vi "IGC100 Close.vi"(2 "error in":errorcluster, 3 "VISA in":refnum<visa-resource-name>) -> (0 "error out":errorcluster)   [LabVIEW 2010]
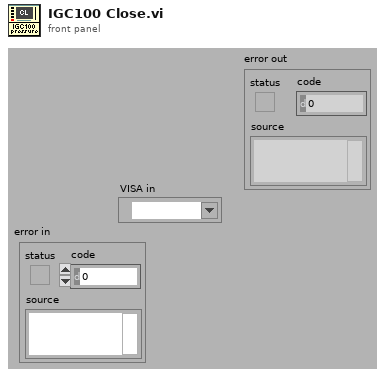
[diagram p1: front panel]
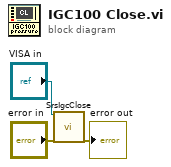
[diagram p0: block diagram]
diagram:
  n1 = call "SrsIgcClose.vi"("VISA session"="VISA in", "error in (no error)"="error in") -> ("error out"=→"error out":errorcluster)  [unwired: 17 in]
